vi "Agilent PWM Measure.vi"(7 "Agilent PWM":T2, 8 "error in (no error)":errorcluster, 11 "VISA Resource Name":refnum<visa-resource-name>) -> (0 "error out":errorcluster {"code" format="%.0x"}, 2 "PWM Measurement":T1 caption="This reading is allways in the base units\ni.e. V, A, Ohms, Hz, Sec, etc." format="%#_10f", 3 "dup VISA Resource Name":refnum<visa-resource-name>)   [LabVIEW 2011]
uses:
  TypeDefs/Agilent PWM Instrument Info.ctl
  PWM Measurement.ctl
  TypeDefs/Agilent PWM Trigger Source.ctl
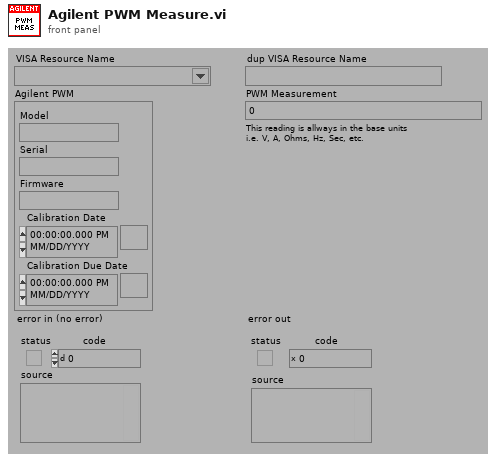
[diagram p1: front panel]
types:
  T1 = typedef "PWM Measurement.ctl" = dbl
  T2 = typedef "Agilent PWM Instrument Info.ctl" = cluster{"Model":string, "Serial":string, "Firmware":string, "Calibration Date":timestamp, "Calibration Due Date":timestamp}
  T3 = typedef "Agilent PWM Trigger Source.ctl" = enum16{"Immediate", "Bus", "Hold", "Internal", "External"}
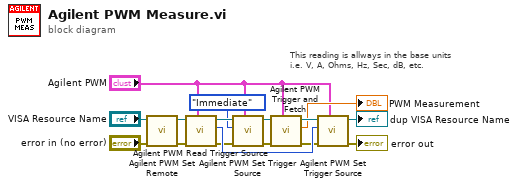
[diagram p0: block diagram]
diagram:
  # "This reading is allways in the base units\ni.e. V, A, Ohms, Hz, Sec, dB, etc."
  n1 = call "Agilent PWM Set Remote.vi"("error in (no error)"="error in (no error)", "VISA Resource Name"="VISA Resource Name") -> ("error out"=w7:errorcluster, "dup VISA Resource Name"=w8:refnum<visa-resource-name>)  [unwired: 8 out]
  n2 = call "Agilent PWM Read Trigger Source.vi"("Agilent PWM"="Agilent PWM", "error in (no error)"=w7, "VISA Resource Name"=w8) -> ("error out"=w3:errorcluster, "Trigger Source"=w14:T3, "dup VISA Resource Name"=w4:refnum<visa-resource-name>)  [unwired: 6 out]
  n3 = call "Agilent PWM Set Trigger Source.vi"("Agilent PWM"="Agilent PWM", "error in (no error)"=w3, "Trigger Source"=Agilent_PWM_Trigger_Source."Immediate", "VISA Resource Name"=w4) -> ("error out"=w6:errorcluster, "dup VISA Resource Name"=w5:refnum<visa-resource-name>)  [unwired: 6 out]
  n4 = call "Agilent PWM Trigger and Fetch.vi"("Agilent PWM"="Agilent PWM", "error in (no error)"=w6, "VISA Resource Name"=w5) -> ("error out"=w13:errorcluster, "Data Reading"=→"PWM Measurement":T1, "dup VISA Resource Name"=w12:refnum<visa-resource-name>)  [unwired: 1 in, 5 out]
  n5 = call "Agilent PWM Set Trigger Source.vi"("Agilent PWM"="Agilent PWM", "error in (no error)"=w13, "Trigger Source"=w14, "VISA Resource Name"=w12) -> ("error out"=→"error out":errorcluster, "dup VISA Resource Name"=→"dup VISA Resource Name":refnum<visa-resource-name>)  [unwired: 6 out]
